vi "Example Callback - AllValues Callback.vi"(4 "AllValues":refnum<user-event>, 5 "Event Data":T1, 6 "Control Ref":refnum<k24>, 7 "Event Common Data":T2) -> ()   [LabVIEW 2013]
uses:
  C:/tf/play/labview/Tinkerforge.dll
  Tinkerforge.dll
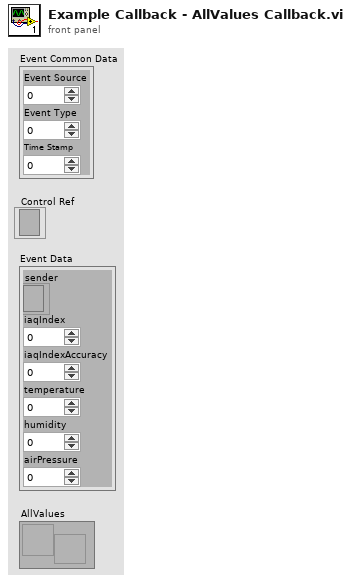
[diagram p1: front panel]
types:
  T1 = cluster{"sender":refnum<k24>, "iaqIndex":i32, "iaqIndexAccuracy":u8, "temperature":i32, "humidity":i32, "airPressure":i32}
  T2 = cluster{"Event Source":i32, "Event Type":u32, "Time Stamp":u32}
  T3 = cluster{"temperature":i32, "humidity":i32, "airPressure":i32, "iaqIndex":i32, "iaqIndexAccuracy":u8}
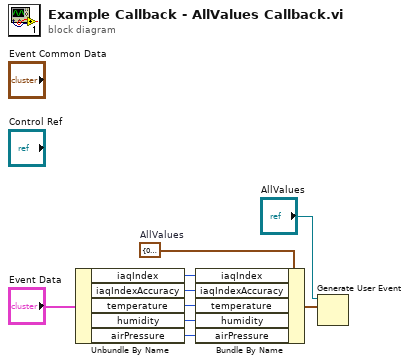
[diagram p0: block diagram]
diagram:
  w8 = T3 {"temperature"=0, "humidity"=0, "airPressure"=0, "iaqIndex"=0, "iaqIndexAccuracy"=0}  # AllValues
  n1 = Unbundle By Name("Event Data") -> ("iaqIndex"=w5:i32, "iaqIndexAccuracy"=w4:u8, "temperature"=w3:i32, "humidity"=w2:i32, "airPressure"=w1:i32)
  n2 = Bundle By Name(cluster=w8, "iaqIndex"=w5, "iaqIndexAccuracy"=w4, "temperature"=w3, "humidity"=w2, "airPressure"=w1) -> (w7:T3)
  n3 = Generate User Event(user event="AllValues", event data cluster=w7) -> ()  [unwired: 2 in, 2 out]
